vi "thcd_get_flow.vi"(6 "err_in":errorcluster, 7 "thcd_visa":refnum<visa-resource-name>, 9 "thcd_ch":T1=enum."1", 10 "thcd_b2r":u32, 11 "thcd_delay":u32=500) -> (0 "thcd_st":bool, 2 "thcd_res_str":string, 3 "thcd_res":T2, 4 "err_out":errorcluster, 5 "thcd_visa":refnum<visa-resource-name>)   [LabVIEW 2020]
uses:
  mks946_controls/ctrl_chn_thcd.ctl
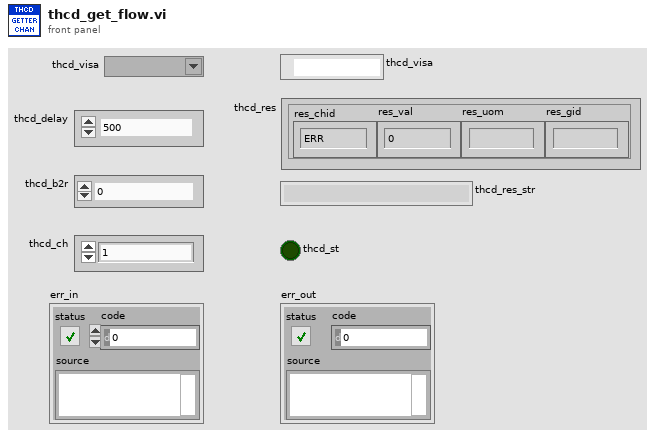
[diagram p1: front panel]
types:
  T1 = typedef "ctrl_chn_thcd.ctl" = enum8{"ERR", "1", "2", "3", "4"}
  T2 = cluster{"res_chid":T1, "res_val":dbl, "res_uom":string, "res_gid":string}
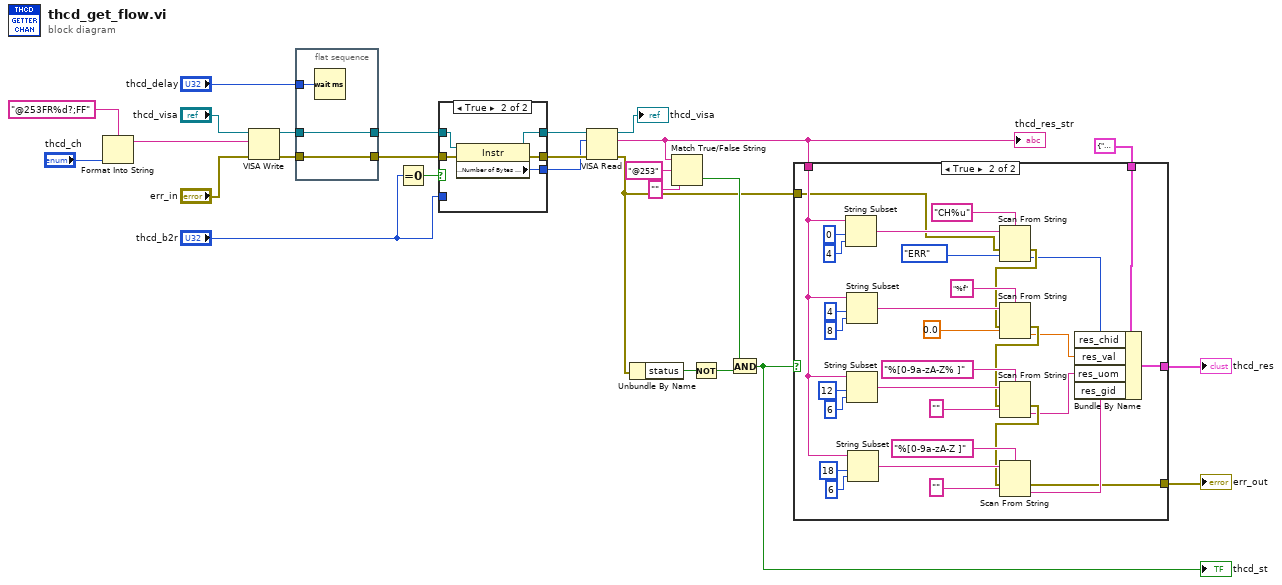
[diagram p0: block diagram]
diagram:
  n1 = Format Into String(format string="@253FR%d?;FF", "thcd_ch") -> (resulting string=w22:string)  [unwired: 2 in, 1 out]
  n2 = VISA Write(VISA resource name="thcd_visa", write buffer=w22, error in (no error)="err_in") -> (VISA resource name out=w26:refnum<visa-resource-name>, error out=w27:errorcluster)  [unwired: 1 out]
  n3 = flat-sequence {
    tunnel: w27 -> [w29]
    tunnel: [w29] -> w10
    tunnel: w26 -> [w28]
    tunnel: [w28] -> w11
    tunnel: "thcd_delay" -> [w30]
    frame #0 {
      n4 = Wait (ms)(milliseconds to wait=w30) -> ()  [unwired: 1 out]
    }
  }
  n5 = Equal To 0?(x="thcd_b2r") -> (x = 0?=w12:bool)
  n6 = case shown="True" w12 {
    tunnel: [w32 w38] -> w9
    tunnel: [w31 w37] -> w8
    tunnel: [w33 w36] -> w7
    tunnel: "thcd_b2r" -> [w33 _]
    tunnel: w11 -> [w32 w35]
    tunnel: w10 -> [w31 w34]
    frame False {
    }
    frame True {
      n7 = property class="Instr"(reference=w35, error in=w34) -> (reference out=w38:refnum<visa-resource-name>, error out=w37:errorcluster, "Serial Settings:Number of Bytes at Serial Port"=w36:u32)
    }
  }
  n8 = VISA Read(VISA resource name=w9, byte count=w7, error in (no error)=w8) -> (VISA resource name out=→"thcd_visa":refnum<visa-resource-name>, read buffer=w18:string, error out=w2:errorcluster)  [unwired: 1 out]
  "thcd_res_str" <- w18
  n9 = Unbundle By Name(w2) -> ("status"=w15:bool)
  n10 = Match True/False String(2:"" ("false string"), 3:"@253" ("true string"), 4:w18) -> (0:w14:bool)  [unwired: 1 out]
  n11 = Not(x=w15) -> (.not. x?=w13:bool)
  n12 = And(x=w14, y=w13) -> (x .and. y?=w1:bool)
  "thcd_st" <- w1
  n13 = case shown="True" w1 {
    tunnel: w18 -> [_ w46]
    tunnel: w2 -> [w40 w45]
    tunnel: [w40 w41] -> w5
    tunnel: T2 {"res_chid"=enum."ERR", "res_val"=0.0, "res_uom"="", "res_gid"=""} ("thcd_res 2") -> [w39 w44]
    tunnel: [w39 w43] -> w3
    frame False {
    }
    frame True {
      n14 = String Subset(string=w46, offset (0)=0, length (rest)=4 ("length (rest)")) -> (substring=w64:string)
      n15 = String Subset(string=w46, offset (0)=4, length (rest)=8 ("length (rest)")) -> (substring=w60:string)
      n16 = String Subset(string=w46, offset (0)=12, length (rest)=6 ("length (rest)")) -> (substring=w57:string)
      n17 = String Subset(string=w46, offset (0)=18, length (rest)=6 ("length (rest)")) -> (substring=w56:string)
      n18 = Scan From String(format string="CH%u", input string=w64, error in=w45, default 1=ctrl_chn_thcd."ERR" ("res_chid")) -> (error out=w52:errorcluster, output 1=w42:T1)  [unwired: 1 in, 2 out]
      n19 = Scan From String(format string="%f", input string=w60, error in=w52, default 1=0.0 ("default value 1")) -> (error out=w51:errorcluster, output 1=w49:dbl)  [unwired: 1 in, 2 out]
      n20 = Scan From String(format string="%[0-9a-zA-Z% ]", input string=w57, error in=w51, default 1="" ("default value 1")) -> (error out=w50:errorcluster, output 1=w48:string)  [unwired: 1 in, 2 out]
      n21 = Scan From String(format string="%[0-9a-zA-Z ]", input string=w56, error in=w50, default 1="" ("default value 1")) -> (error out=w41:errorcluster, output 1=w47:string)  [unwired: 1 in, 2 out]
      n22 = Bundle By Name(cluster=w44, "res_chid"=w42, "res_val"=w49, "res_uom"=w48, "res_gid"=w47) -> (w43:T2)
    }
  }
  "err_out" <- w5
  "thcd_res" <- w3
